vi "Shrink Pixel Map.vi"(9 "Flipped?":bool, 10 "Shrink Factor  (0.5-1)":dbl=0.5 min=0.5 max=1.0, 11 "Pixel Map IN":i32[](array[numeric])=[-43, -42, -41, -40, -39, -38, -37, -36, -35, -34, -33, -32, -31, -30, -29, -28, -27, -26, -25, -24, -23, -22, -21, -20, -19, -18, -17, -16, -15, -14, -13, -12, -11, -10, -9, -8, -7, -6, -5, -4, -3, -2, -1, 0, 1, 2, 3, 4, 5, 6, 7, 8, 9, 10, 11, 12, 13, 14, 15, 16, 17, 18, 19, 20, 21, 22, 23, 24, 25, 26, 27, 28, 29, 30, 31, 32, 33, 34, 35, 36, 37, 38, 39, 40, 41, 42, 43, 44, 45, 46, 47, 48, 49, 50, 51, 52, 53, 54, 55, 56, 57, 58, 59, 60, 61, 62, 63, 64, 65, 66, 67, 68, 69, 70, 71, 72, 73, 74, 75, 76, 77, 78, 79, 80, 81, 82, 83, 84, 85, 86, 87, 88, 89, 90, 91, 92, 93, 94, 95, 96, 97, 98, 99, 100, 101, 102, 103, 104, 105, 106, 107, 108, 109, 110, 111, 112, 113, 114, 115, 116, 117, 118, 119, 120, 121, 122, 123, 124, 125, 126, 127, 128, 129, 130, 131, 132, 133, 134, 135, 136, 137, 138, 139, 140, 141, 142, 143, 144, 145, 146, 147, 148, 149, 150, 151, 152, 153, 154, 155, 156, 157, 158, 159, 160, 161, 162, 163, 164, 165, 166, 167, 168, 169, 170, 171, 172, 173, 174, 175, 176, 177, 178, 179, 180, 181, 182, 183, 184, 185, 186, 187, 188, 189, 190, 191, 192, 193, 194, 195, 196, 197, 198, 199, 200, 201, 202, 203, 204, 205, 206, 207, 208, 209, 210, 211, 212, 213, 214, 215, 216, 217, 218, 219, 220, 221, 222, 223, 224, 225, 226, 227, 228, 229, 230, 231, 232, 233, 234, 235, 236, 237, 238, 239, 240, 241, 242, 243, 244, 245, 246, 247, 248, 249, 250, 251, 252, 253, 254, 255, 256, 257, 258, 259, 260, 261, 262, 263, 264, 265, 266, 267, 268, 269, 270, 271, 272, 273, 274, 275, 276, 277, 278, 279, 280, 281, 282, 283, 284, 285, 286, 287, 288, 289, 290, 291, 292, 293, 294, 295, 296, 297, 298, 299, 300, 301, 302, 303, 304, 305, 306, 307, 308, 309, 310, 311, 312, 313, 314, 315, 316, 317, 318, 319, 320, 321, 322, 323, 324, 325, 326, 327, 328, 329, 330, 331, 332, 333, 334, 335, 336, 337, 338, 339, 340, 341, 342, 343, 344, 345, 346, 347, 348, 349, 350, 351, 352, 353, 354, 355, 356, 357, 358, 359, 360, 361, 362, 363, 364, 365, 366, 367, 368, 369, 370, 371, 372, 373, 374, 375, 376, 377, 378, 379, 380, 381, 382, 383, 384, 385, 386, 387, 388, 389, 390, 391, 392, 393, 394, 395, 396, 397, 398, 399, 400, 401, 402, 403, 404, 405, 406, 407, 408, 409, 410, 411, 412, 413, 414, 415, 416, 417, 418, 419, 420, 421, 422, 423, 424, 425, 426, 427, 428, 429, 430, 431, 432, 433, 434, 435, 436, 437, 438, 439, 440, 441, 442, 443, 444, 445, 446, 447, 448, 449, 450, 451, 452, 453, 454, 455, 456, 457, 458, 459, 460, 461, 462, 463, 464, 465, 466, 467, 468]) -> (1 "Excess pixels (Right)":i32, 2 "Excess pixels (Left)":i32, 3 "pixel map OUT (Zoomed out)":i32[](array[numeric]))   [LabVIEW 2012]
panel:
  out "Points of shrinkage":cluster{i32[], i32[]}(graph)
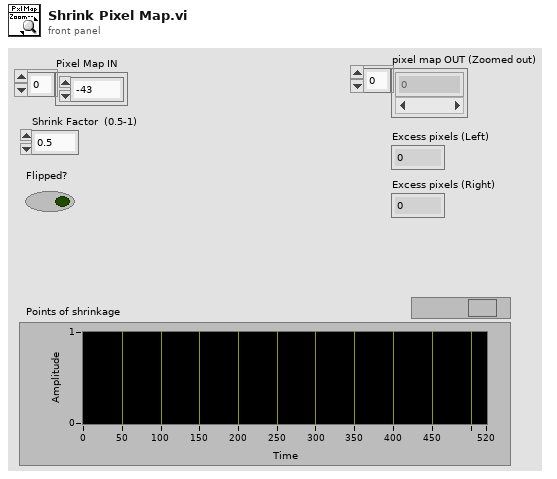
[diagram p1: front panel]
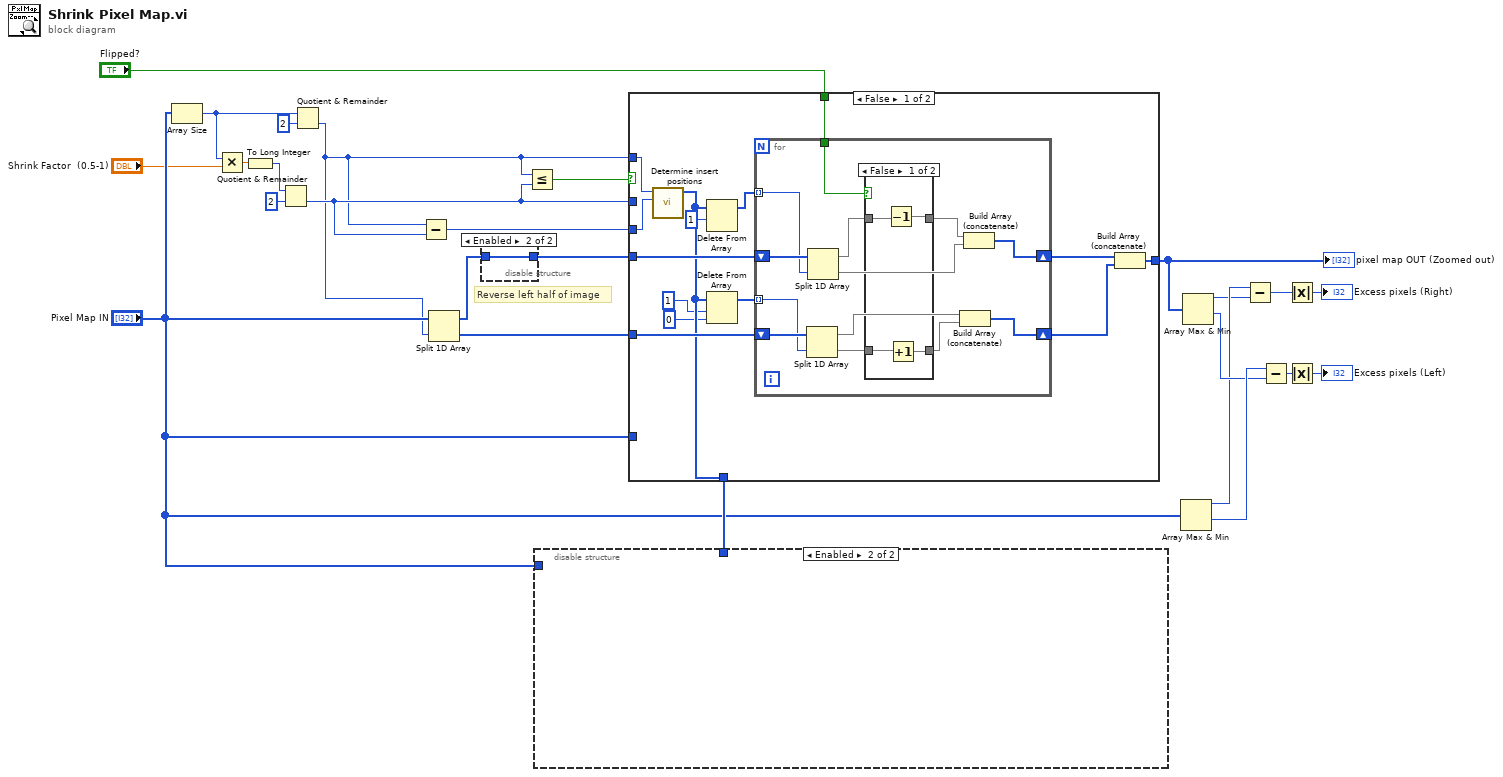
[diagram p0: block diagram]
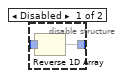
[diagram p2: hidden frame]
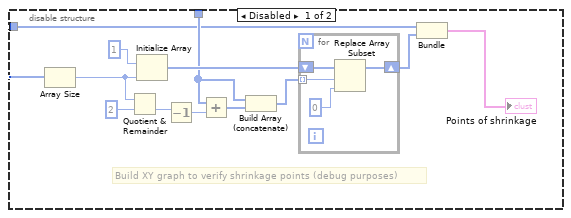
[diagram p3: hidden frame]
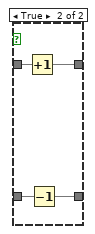
[diagram p4: hidden frame]
diagram:
  # "Reverse left half of image"
  n1 = Array Size(array="Pixel Map IN") -> (size(s)=w17:i32)
  n2 = Multiply(x=w17, y="Shrink Factor  (0.5-1)") -> (x*y=w24:dbl)
  n3 = To Long Integer(number=w24) -> (32bit integer=w22:i32)
  n4 = Quotient & Remainder(x=w22, y=2) -> (floor(x/y)=w5:i32)  [unwired: 1 out]
  n5 = Quotient & Remainder(x=w17, y=2) -> (floor(x/y)=w4:i32)  [unwired: 1 out]
  n6 = Subtract(x=w4, y=w5) -> (x-y=w3:i32)
  n7 = Split 1D Array(array="Pixel Map IN", index=w4) -> (first subarray=w20:i32[], second subarray=w18:i32[])
  n8 = disable-structure shown="Enabled" {
    disable-tunnel: w20 -> [w27 w28]
    disable-tunnel: [w26 w28] -> w19
    frame Disabled {
      n9 = Reverse 1D Array(array=w27) -> (reversed array=w26:i32[])
    }
    frame Enabled {
    }
  }
  n10 = Less Or Equal?(x=w4, y=w5) -> (x <= y?=w21:bool)
  n11 = case shown="False" w21 {
    tunnel: w4 -> [w42 _]
    tunnel: w5 -> [_ _]
    tunnel: w19 -> [w41 _]
    tunnel: w18 -> [w40 _]
    tunnel: [w37 w64] -> w9
    tunnel: "Pixel Map IN" -> [_ w64]
    tunnel: [w32 _] -> w8
    tunnel: w3 -> [w36 _]
    tunnel: "Flipped?" -> [w35 _]
    frame False {
      n12 = call "Determine insert positions.vi"("Points to be distributed (D)"=w36, "Array size (N)"=w42) -> ("Distribution Indices (with one extra) - delete required end"=w32:i32[])  [unwired: 8 in, 1 out]
      n13 = Delete From Array(array=w32, length=1) -> (array with subset deleted=w33:i32[])  [unwired: 1 in, 1 out]
      n14 = Delete From Array(array=w32, length=1, index=0) -> (array with subset deleted=w29:i32[])  [unwired: 1 out]
      n15 = for {
        tunnel: w33 -> [w48] mode=indexing
        shift-right: [w53] -> w39
        shift-left: w41 -> [w55]
        shift-right: [w47] -> w38
        shift-left: w40 -> [w49]
        tunnel: w29 -> [w44] mode=indexing
        tunnel: w35 -> [w43]
        n16 = Split 1D Array(array=w49, index=w44) -> (first subarray=w51:i32[], second subarray=w50:i32[])
        n17 = Split 1D Array(array=w55, index=w48) -> (first subarray=w46:i32[], second subarray=w54:i32[])
        n18 = case shown="False" w43 {
          tunnel: [w56 w63] -> w52
          tunnel: w50 -> [w57 w62]
          tunnel: w46 -> [w59 w61]
          tunnel: [w58 w60] -> w45
          frame False {
            n19 = Decrement(x=w59) -> (x-1=w58:i32[])
            n20 = Increment(x=w57) -> (x+1=w56:i32[])
          }
          frame True {
            n21 = Increment(x=w61) -> (x+1=w60:i32[])
            n22 = Decrement(x=w62) -> (x-1=w63:i32[])
          }
        }
        n23 = Build Array (concatenate)(w51, w52) -> (w47:i32[])
        n24 = Build Array (concatenate)(w45, w54) -> (w53:i32[])
      }
      n25 = Build Array (concatenate)(w39, w38) -> (w37:i32[])
    }
    frame True {
      # "Same size... do nothing!!"
    }
  }
  "pixel map OUT (Zoomed out)" <- w9
  n26 = disable-structure shown="Enabled" {
    disable-tunnel: w8 -> [w72 _]
    disable-tunnel: "Pixel Map IN" -> [w66 _]
    frame Disabled {
      # "Build XY graph to verify shrinkage points (debug purposes)"
      n27 = Array Size(array=w66) -> (size(s)=w65:i32)
      n28 = Quotient & Remainder(x=w65, y=2) -> (floor(x/y)=w68:i32)  [unwired: 1 out]
      n29 = Initialize Array(1, w65) -> (w74:i32[])
      n30 = Decrement(x=w68) -> (x-1=w67:i32)
      n31 = Add(x=w72, y=w67) -> (x+y=w71:i32[])
      n32 = Build Array (concatenate)(w72, w71) -> (w70:i32[])
      n33 = for {
        tunnel: w70 -> [w79] mode=indexing
        shift-right: [w77] -> w75
        shift-left: w74 -> [w80]
        n34 = Replace Array Subset(array=w80, new element=0 ("new element/subarray"), index=w79) -> (w77:i32[])
      }
      n35 = Bundle("Pixel Map IN"=w66, w75) -> (→"Points of shrinkage":cluster{"Pixel Map IN":i32[], i32[]})  [unwired: 1 in]
    }
    frame Enabled {
    }
  }
  n36 = Array Max & Min(array="Pixel Map IN") -> (max value=w11:i32, min value=w15:i32)  [unwired: 2 out]
  n37 = Array Max & Min(array=w9) -> (max value=w10:i32, min value=w14:i32)  [unwired: 2 out]
  n38 = Subtract(x=w11, y=w10) -> (x-y=w16:i32)
  n39 = Subtract(x=w15, y=w14) -> (x-y=w13:i32)
  n40 = Absolute Value(x=w16) -> (abs(x)=→"Excess pixels (Right)":i32)
  n41 = Absolute Value(x=w13) -> (abs(x)=→"Excess pixels (Left)":i32)
